vi "Set Testing State.vi"(8 "error in (no error)":errorcluster, 11 "Testing State":bool) -> (0 "error out":errorcluster)   [LabVIEW 2018]
doc: "This subVI enqueues the named action in to the communications queue along with the input data."
uses:
  Private Controls/Module Action.ctl
  File IO.lvlib
  Private Controls/Module Data.ctl
panel:
  in  "Action":T1=enum."Set Testing State"
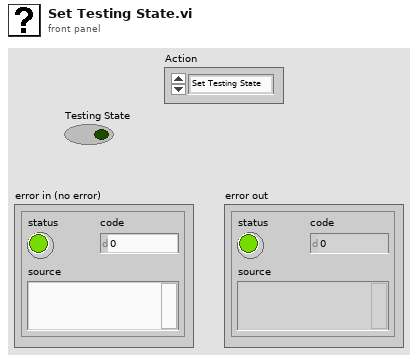
[diagram p1: front panel]
types:
  T1 = typedef "File IO.lvlib/Module Action.ctl" = enum8{"Timeout", "Continue Test", "Init", "Error", "Exit", "Save Calibration Data", "Save Accel Data", "Set Testing State", "Set Recording State", "Set Test Information", "Close Data File", "Add to System Log", "Save Stored APU Data", "Load APU Setup File", "Increment Run Count", "Write To Report", "Flush TDMS to File", "Change TDMS Group Name"}
  T2 = typedef "File IO.lvlib/Module Data.ctl" = cluster{"Data":variant, "Action":T3}
  T3 = typedef "File IO.lvlib/Module Action.ctl" = enum8{"Timeout", "Continue Test", "Init", "Error", "Exit", "Save Calibration Data", "Save Accel Data", "Set Recording State", "Set Test Information", "Write to System Log", "Save Stored APU Data", "Load APU Setup File", "Increment Run Count", "Write To Report"}
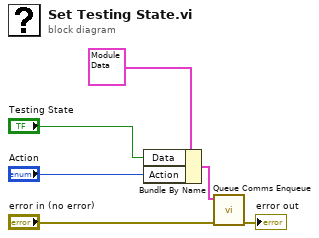
[diagram p0: block diagram]
diagram:
  n1 = Bundle By Name(cluster=T2 {"Data"=variant, "Action"=enum."Init"} ("element"), "Data"="Testing State", "Action"="Action") -> (w5:T2)
  n2 = call "Queue Comms Enqueue.vi"("error in (no error)"="error in (no error)", "element"=w5) -> ("error out"=→"error out":errorcluster)  [unwired: 9 in]
